vi "Test_Hysteresis_max.vi"() -> ()   [LabVIEW 2022 SP3]
panel:
  in  "stop":bool
  out "Deviation":bool
  in  "Max":dbl=26.0 format="%#_13g"
  in  "H":dbl=22.0 format="%#_13g"
  in  "input (-)":dbl
  in  "input(+)":dbl
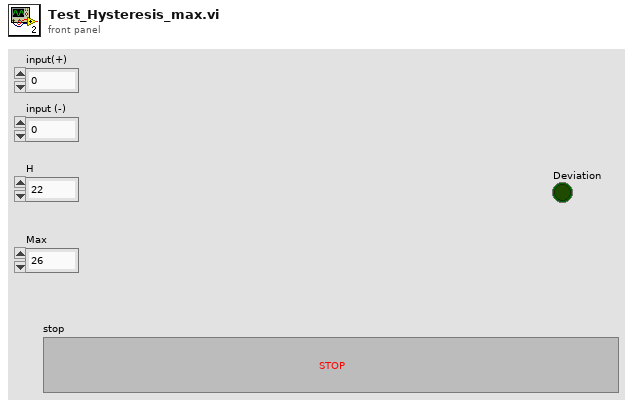
[diagram p1: front panel]
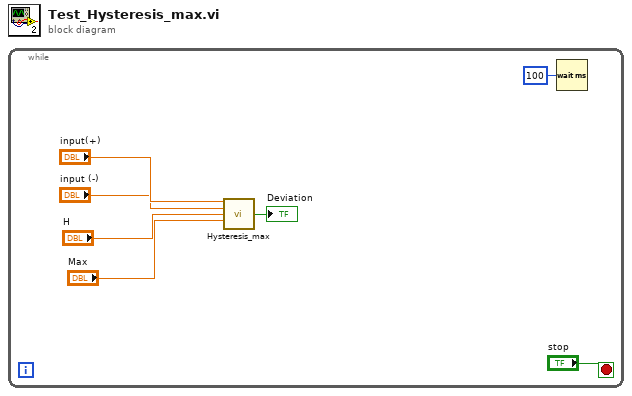
[diagram p0: block diagram]
diagram:
  n1 = while {
    stop <- "stop" stop-if-true
    n2 = call "Hysteresis_max.vi"("input(+)"="input(+)", "input (-)"="input (-)", "H"="H", "Max"="Max") -> ("Deviation"=→"Deviation":bool)  [unwired: 10 in, 1 out]
    n3 = Wait (ms)(milliseconds to wait=u32 100) -> ()  [unwired: 1 out]
  }
